vi "database reuse unit tests.vi"() -> ()   [LabVIEW 2020]
uses:
  Database Reuse.lvlib
panel:
  out "VCluster out 3":variant
  out "VCluster Columns 3":string[](array[string])
  out "VCluster out 2":variant
  out "VCluster Columns 2":string[](array[string])
  out "VCluster Columns":string[](array[string])
  out "VCluster out":variant
  out "data (Cluster) 3":variant
  out "data (Cluster) 2":variant
  out "data (Cluster)":variant
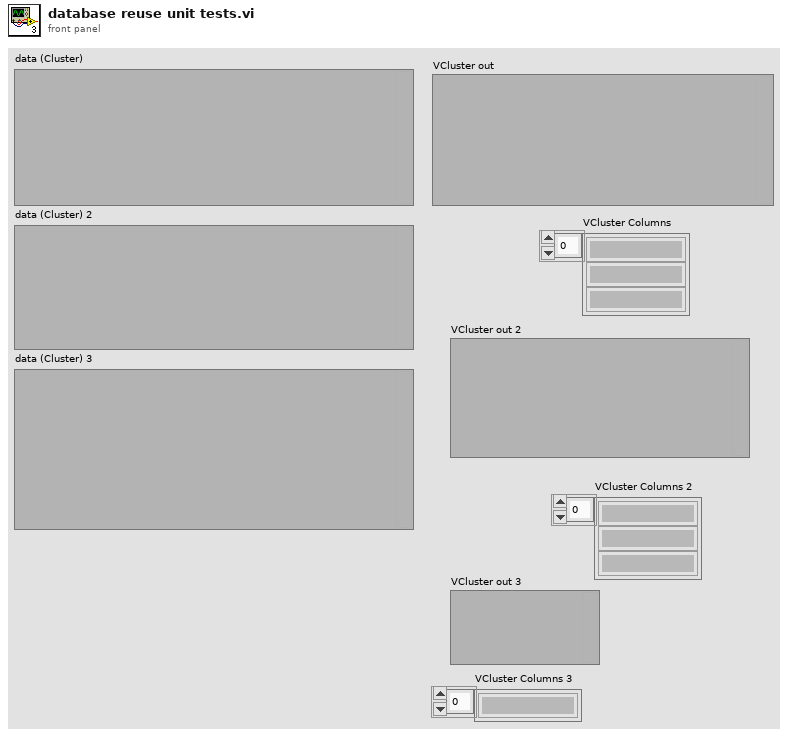
[diagram p1: front panel]
types:
  T1 = cluster{"test":string, "test2":dbl, "test3":timestamp}
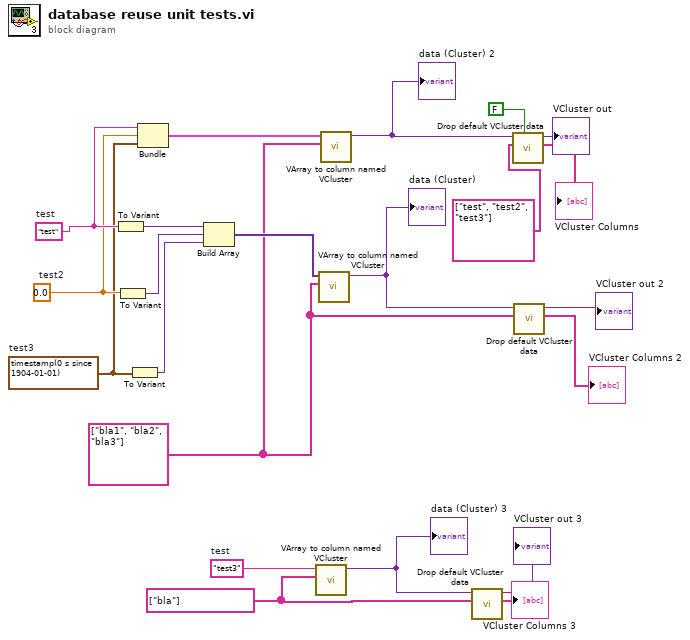
[diagram p0: block diagram]
diagram:
  w3 = string[] ["bla"] ("columns")
  w14 = "test3"  # test
  w7 = string[] ["bla1", "bla2", "bla3"]
  w16 = timestamp(0 s since 1904-01-01)  # test3
  w17 = 0.0  # test2
  w18 = "test"  # test
  n1 = To Variant(anything=w18) -> (Variant=w22:variant)
  n2 = To Variant(anything=w17) -> (Variant=w21:variant)
  n3 = To Variant(anything=w16) -> (Variant=w20:variant)
  n4 = Bundle("test"=w18, "test2"=w17, "test3"=w16) -> (w15:T1)  [unwired: 1 in]
  n5 = Build Array(w22, w21, w20) -> (w19:variant[])
  n6 = call "VArray to column named VCluster.vi"("columns"=w3, "data"=w14) -> ("data (Cluster)"=w4:variant)  [unwired: 8 in, 1 out]
  "data (Cluster) 3" <- w4
  n7 = call "VArray to column named VCluster.vi"("columns"=w7, "data"=w19) -> ("data (Cluster)"=w8:variant)  [unwired: 8 in, 1 out]
  "data (Cluster)" <- w8
  n8 = call "VArray to column named VCluster.vi"("columns"=w7, "data"=w15) -> ("data (Cluster)"=w13:variant)  [unwired: 8 in, 1 out]
  "data (Cluster) 2" <- w13
  n9 = call "Drop default VCluster data.vi"("Columns"=w3, "VCluster in"=w4) -> ("VCluster Columns"=→"VCluster Columns 3":string[], "VCluster out"=→"VCluster out 3":variant)  [unwired: 7 in, 1 out]
  n10 = call "Drop default VCluster data.vi"("Drop default numeric? (F)"=FALSE, "Columns"=string[] ["test", "test2", "test3"], "VCluster in"=w13) -> ("VCluster Columns"=→"VCluster Columns":string[], "VCluster out"=→"VCluster out":variant)  [unwired: 6 in, 1 out]
  n11 = call "Drop default VCluster data.vi"("Columns"=w7, "VCluster in"=w8) -> ("VCluster Columns"=→"VCluster Columns 2":string[], "VCluster out"=→"VCluster out 2":variant)  [unwired: 7 in, 1 out]
